vi "tempcondsetpt.vi"(1 "Set Point":dbl=77.0 format="%.2f", 2 "error in":errorcluster, 3 "GPIB Address":string="16") -> (0 "error out":errorcluster)   [LabVIEW 2013]
panel:
  # "Set Point for Conductus"
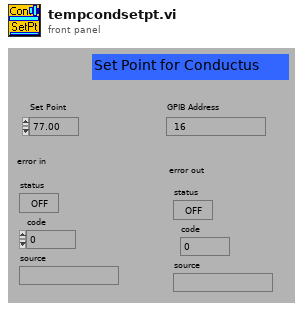
[diagram p1: front panel]
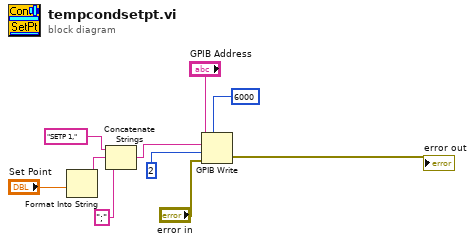
[diagram p0: block diagram]
diagram:
  n1 = Format Into String("Set Point") -> (resulting string=w9:string)  [unwired: 3 in, 1 out]
  n2 = Concatenate Strings("SETP 1,", w9, ";") -> (w1:string)
  n3 = GPIB Write(0:"GPIB Address", 1:w1, 2:2, 3:"error in", 4:6000) -> (6:→"error out":errorcluster)  [unwired: 1 out]
